vi "Matlab.vi"() -> ()   [LabVIEW 2016]
uses:
  <vilib>/Analysis/Matrix/Numeric/Conversions/Array To Matrix - RA2.vi
  <vilib>/Analysis/Matrix/Numeric/Conversions/Matrix To Array - RM.vi
  database/database.lvlib
  <vilib>/Analysis/Matrix/NI_Matrix.lvlib
panel:
  out "element":dbl
  out "Real 2D Array":dbl[][](array[numeric])
  out "2-D Array of Real":dbl[][](array[numeric])
  out "Real":dbl
  out "错误输出":errorcluster
  out "Data 3":string[][](array[string])
  out "Data 2":string[][](array[string])
  out "offset past number":i32
  out "String":string
  out "Data":string[][](array[string])
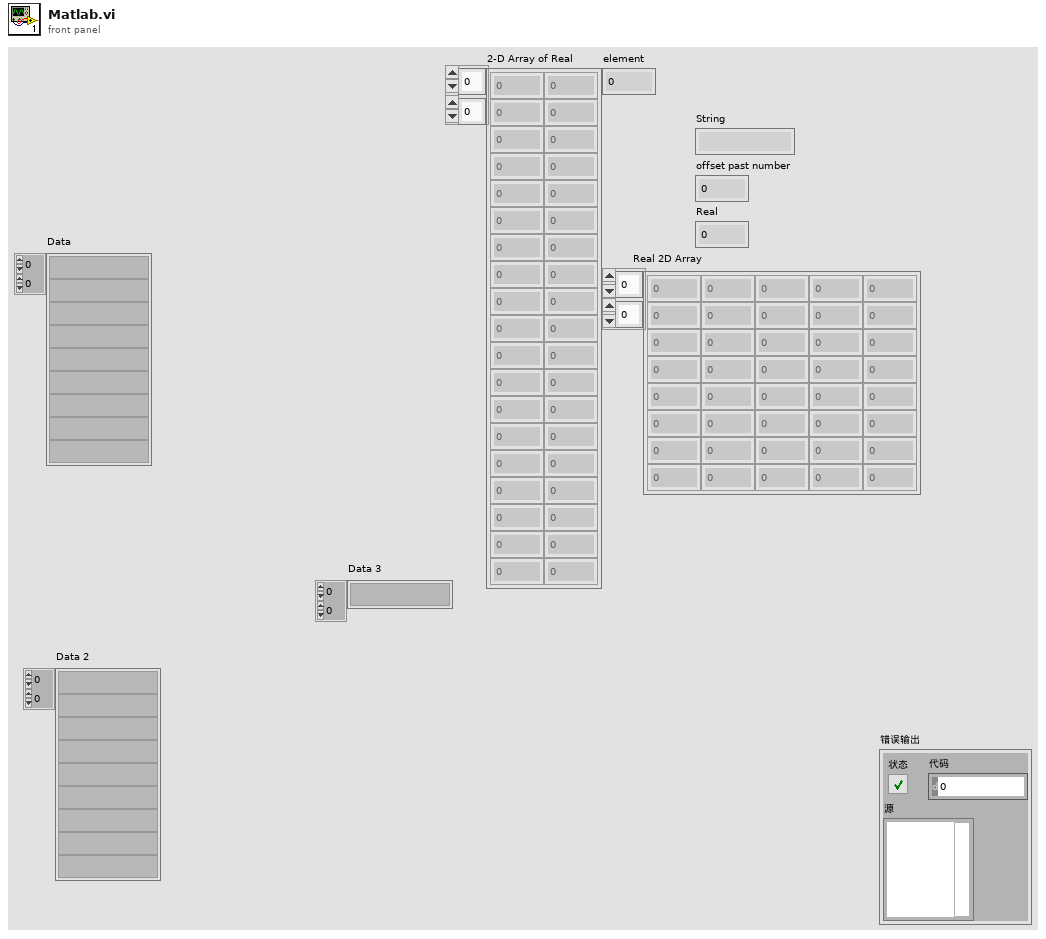
[diagram p1: front panel]
types:
  T1 = typedef "NI_Matrix.lvlib/RealMatrix.ctl" = dbl[][]
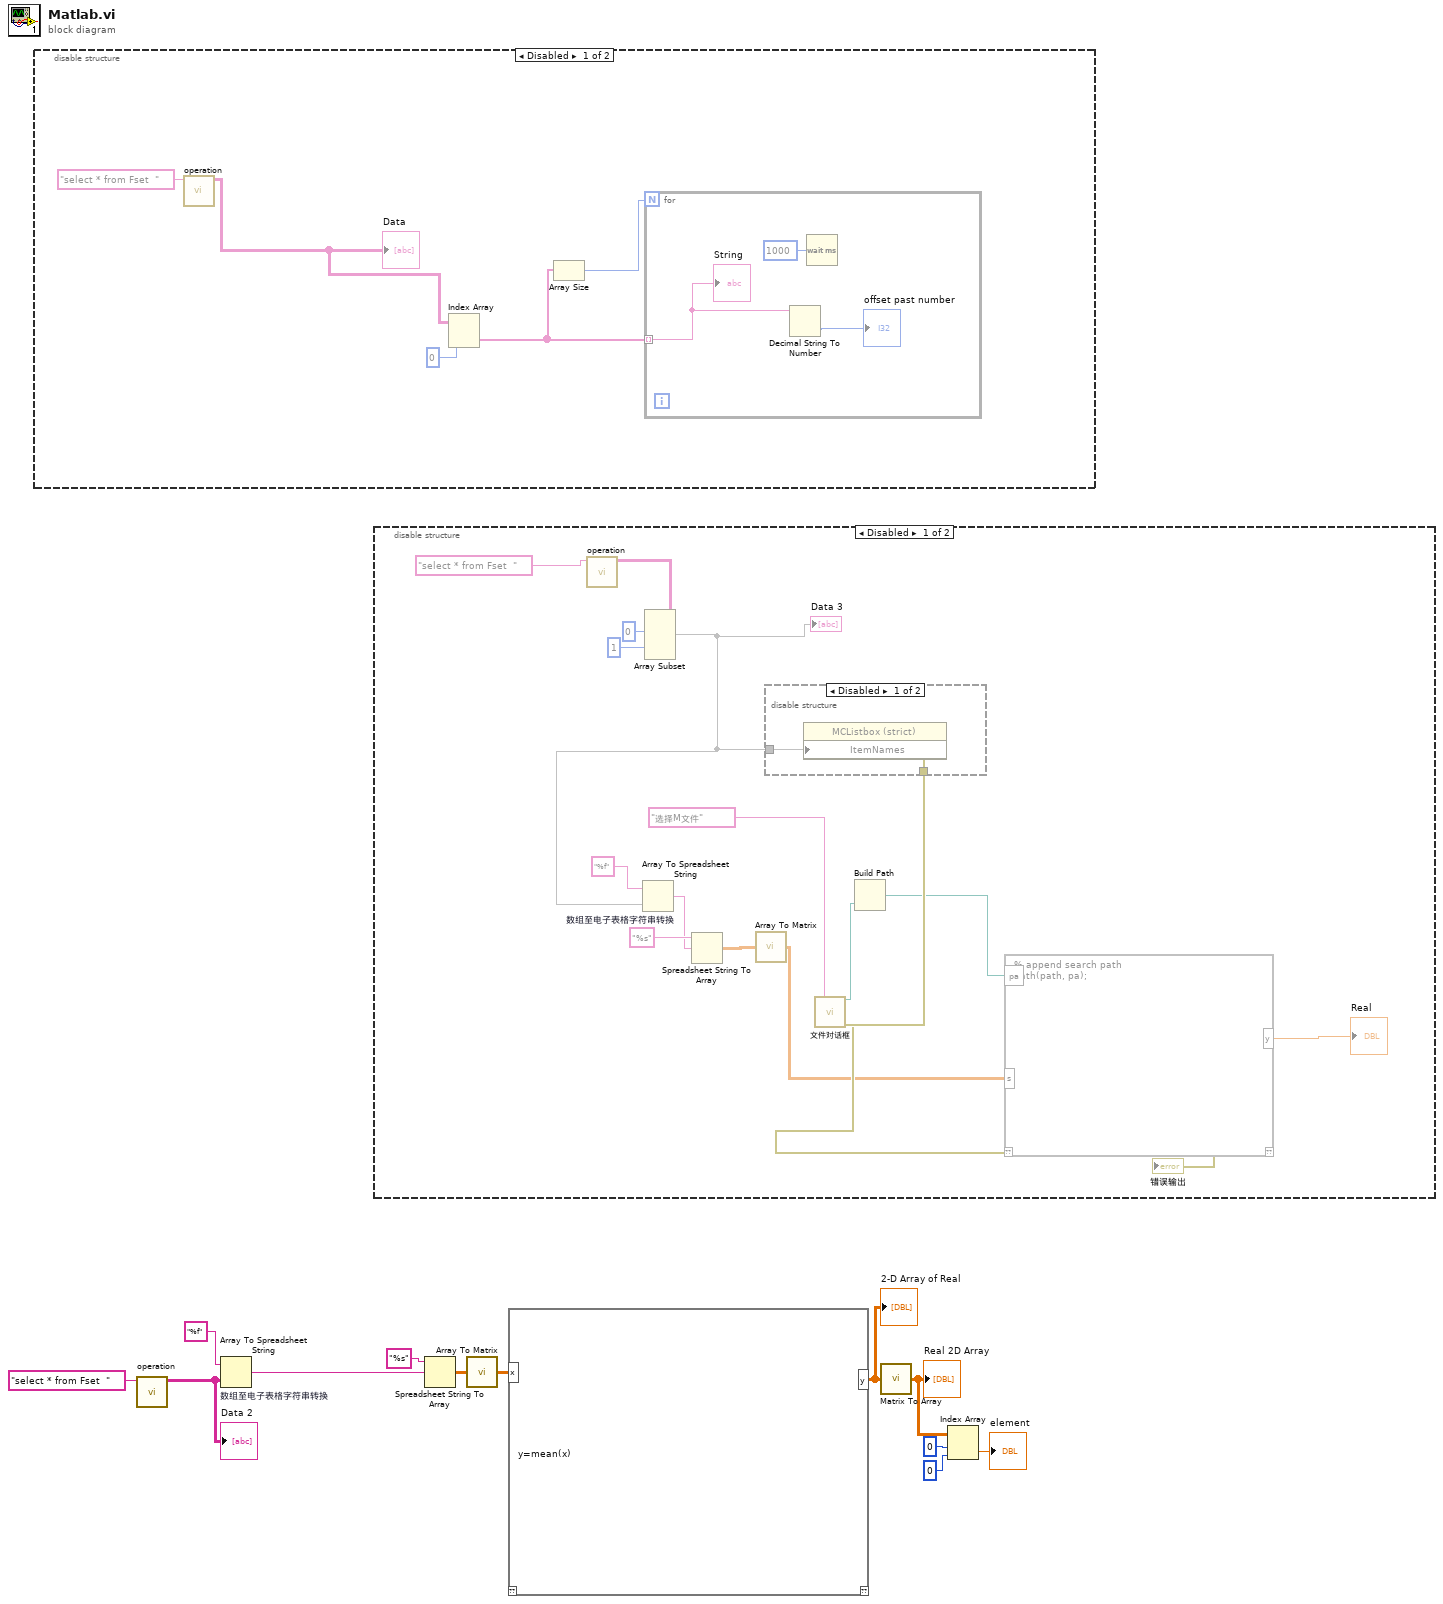
[diagram p0: block diagram]
diagram:
  n1 = disable-structure shown="Disabled" {
    frame Disabled {
      n2 = call "operation.vi"("Command Text"="select * from Fset  ") -> ("Data"=w16:string[][])  [unwired: 9 in]
      "Data" <- w16
      n3 = Index Array(array=w16, index (col)=0 ("disabled index (col)")) -> (element=w13:string[])  [unwired: 1 in]
      n4 = Array Size(array=w13) -> (size(s)=w14:i32)
      n5 = for {
        N: w14 -> [_]
        tunnel: w13 -> [w19] mode=indexing
        n6 = Decimal String To Number(string=w19) -> (number=→"offset past number":i32)  [unwired: 2 in, 1 out]
        n7 = Wait (ms)(milliseconds to wait=u32 1000) -> ()  [unwired: 1 out]
        "String" <- w19
      }
    }
    frame Enabled {
    }
  }
  n8 = call "operation.vi"("Command Text"="select * from Fset  ") -> ("Data"=w7:string[][])  [unwired: 9 in]
  "Data 2" <- w7
  n9 = Array To Spreadsheet String "数组至电子表格字符串转换"(array=w7, 3:"%f" ("格式字符串")) -> (spreadsheet string=w11:string)  [unwired: 1 in]
  n10 = disable-structure shown="Disabled" {
    frame Disabled {
      n11 = call "operation.vi"("Command Text"="select * from Fset  ") -> ("Data"=w36:string[][])  [unwired: 9 in]
      n12 = Array Subset(array=w36, index (row)=0 ("index"), index (col)=1 ("index")) -> (w33:string[][])  [unwired: 2 in]
      "Data 3" <- w33
      n13 = Array To Spreadsheet String "数组至电子表格字符串转换"(array=w33, 3:"%f" ("格式字符串")) -> (spreadsheet string=w29:string)  [unwired: 1 in]
      n14 = Spreadsheet String To Array(format string="%s" ("格式字符串"), spreadsheet string=w29) -> (array=w30:dbl[][])  [unwired: 2 in]
      n15 = call-poly <vilib>:"Array To Matrix.vi"("Real 2D Array"=w30) -> ("Real Matrix"=w24:T1)
      n16 = disable-structure shown="Disabled" {
        disable-tunnel: [w39 _] -> w37
        disable-tunnel: w33 -> [w38 _]
        frame Disabled {
          n17 = property on="Property Node" class="MCListbox (strict)"("ItemNames"=w38) -> (error out=w39:errorcluster)  [unwired: 2 in, 1 out]
        }
        frame Enabled {
        }
      }
      n18 = call "文件对话框"("prompt"="选择M文件", "error in"=w37) -> ("selected path"=w27:path, "error out"=w25:errorcluster)  [unwired: 10 in, 2 out]
      n19 = Build Path(name or relative path=w27) -> (appended path=w26:path)  [unwired: 1 in]
      n20 = script code="% append search path\npath(path, pa);"("??"=w25, "pa"=w26, "s"=w24) -> ("??"=→"错误输出":errorcluster, "y"=→"Real":dbl)
    }
    frame Enabled {
    }
  }
  n21 = Spreadsheet String To Array(format string="%s" ("格式字符串"), spreadsheet string=w11) -> (array=w10:dbl[][])  [unwired: 2 in]
  n22 = call-poly <vilib>:"Array To Matrix.vi"("Real 2D Array"=w10) -> ("Real Matrix"=w6:T1)
  n23 = script code="y=mean(x)"("x"=w6) -> ("y"=w5:dbl[][])  [unwired: 1 in, 1 out]
  "2-D Array of Real" <- w5
  n24 = call-poly <vilib>:"Matrix To Array.vi"("Real Matrix"=w5) -> ("Real 2D Array"=w4:dbl[][])
  "Real 2D Array" <- w4
  n25 = Index Array(array=w4, index (row)=0, index (col)=0 ("disabled index (col)")) -> (element=→"element":dbl)
